vi "Create Channel.vi"   [LabVIEW 2009, in "MicroDAQ.lvlib"]
doc: "Creates a channels to generate or measure signals. This VI is polimorphic."
uses:
  <instrlib>/MicroDAQ/MicroDAQ.lvlib
  <instrlib>/MicroDAQ/Channel/Analog Input/Analog Input.lvclass
  <instrlib>/MicroDAQ/Channel/Analog Output/Analog output.lvclass
  <instrlib>/MicroDAQ/Channel/Digital Input/Digital Input.lvclass
  <instrlib>/MicroDAQ/Channel/Digital output/Digital output.lvclass
  <instrlib>/MicroDAQ/Channel/DSP/DSP.lvclass
  <instrlib>/MicroDAQ/Channel/Encoder/Encoder.lvclass
  <instrlib>/MicroDAQ/Channel/PWM/PWM.lvclass
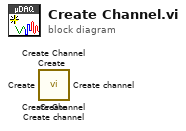
[diagram p0: block diagram]
diagram:
  n1 = call <instrlib>:"Create.vi"() -> ()  [unwired: 10 in, 2 out]
  n2 = call <instrlib>:"Create.vi"() -> ()  [unwired: 10 in, 2 out]
  n3 = call <instrlib>:"Create.vi"() -> ()  [unwired: 10 in, 2 out]
  n4 = call <instrlib>:"Create channel.vi"() -> ()  [unwired: 10 in, 2 out]
  n5 = call <instrlib>:"Create channel.vi"() -> ()  [unwired: 10 in, 2 out]
  n6 = call <instrlib>:"Create Channel.vi"() -> ()  [unwired: 10 in, 2 out]
  n7 = call <instrlib>:"Create Channel.vi"() -> ()  [unwired: 10 in, 2 out]
